vi "clFile_readStr.vi"(7 "length":i32, 8 "offset (0)":i32, 10 "clFile.lvclass":refnum<class "clFile.lvclass">) -> (2 "substring":string)   [LabVIEW 2020, in "vi_lib.lvlib" / "clFile.lvclass"]
uses:
  clFile.lvclass
  clFile.lvclass/clFile.ctl
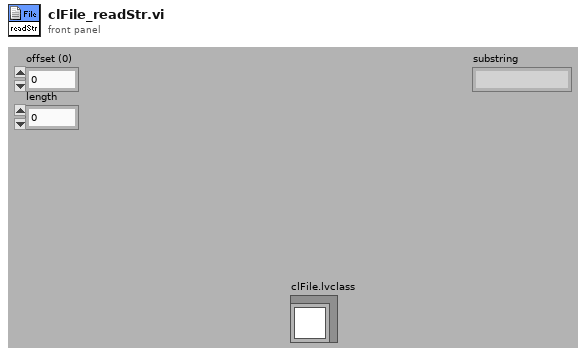
[diagram p1: front panel]
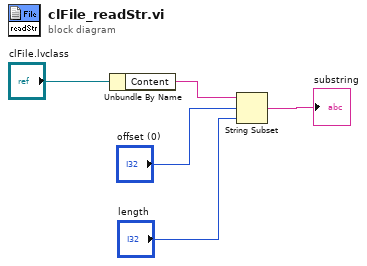
[diagram p0: block diagram]
diagram:
  n1 = Unbundle By Name("clFile.lvclass") -> ("Content"=w4:string)
  n2 = String Subset(string=w4, offset (0)="offset (0)", length (rest)="length") -> (substring=→"substring":string)
